vi "WPI_SwitchOpen.vi"   [LabVIEW 2017]
doc: "Creates a switch reference to the digital input you specify. You must open a reference before using any other VIs on this palette.\n\nThis software is licensed. Open the labview\\readme\\WPI Robotics Library Open Source License.txt file for more information."
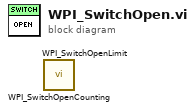
[diagram p0: block diagram]
diagram:
  n1 = call <vilib>:"WPI_SwitchOpenCounting.vi"() -> ()  [unwired: 10 in, 2 out]
  n2 = call <vilib>:"WPI_SwitchOpenLimit.vi"() -> ()  [unwired: 10 in, 2 out]
